vi "Img Plot Frame.vi"(8 "error in (no error)":errorcluster, 9 "frames":T2, 10 "Img Data indexed":cluster{"image data":T1, "bitmap":u32[][]}, 11 "LF2R IDE in":refnum<class "Main Panel.lvclass">) -> (0 "error out":errorcluster, 3 "LF2R IDE out":refnum<class "Main Panel.lvclass">)   [LabVIEW 2018, in "Main Panel.lvlib" / "Main Panel.lvclass"]
uses:
  Main Panel.lvclass
  Image Json Parser/Img Json Frames.ctl
  <vilib>/picture/picture.llb/imagedata.ctl
  Main Panel.lvclass/Main Panel.ctl
  <vilib>/picture/picture.llb/Draw True-Color Pixmap.vi
  Picture Process/Picture Process.lvclass
  Image Json Parser/Image Json Parser.lvclass
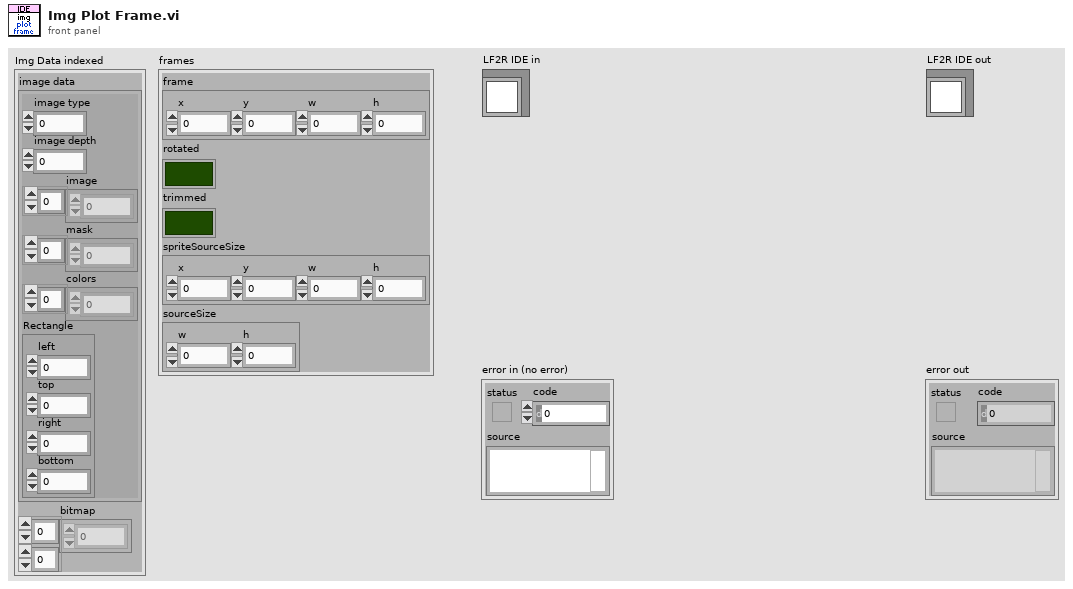
[diagram p1: front panel]
types:
  T1 = typedef "imagedata.ctl" = cluster{"image type":i32, "image depth":i32, "image":u8[], "mask":u8[], "colors":u32[], "Rectangle":cluster{"left":i16, "top":i16, "right":i16, "bottom":i16}}
  T2 = typedef "Image Json Parser.lvclass/Img Json Frames.ctl" = cluster{"frame":cluster{"x":i32, "y":i32, "w":i32, "h":i32}, "rotated":bool, "trimmed":bool, "spriteSourceSize":cluster{"x":i32, "y":i32, "w":i32, "h":i32}, "sourceSize":cluster{"w":i32, "h":i32}}
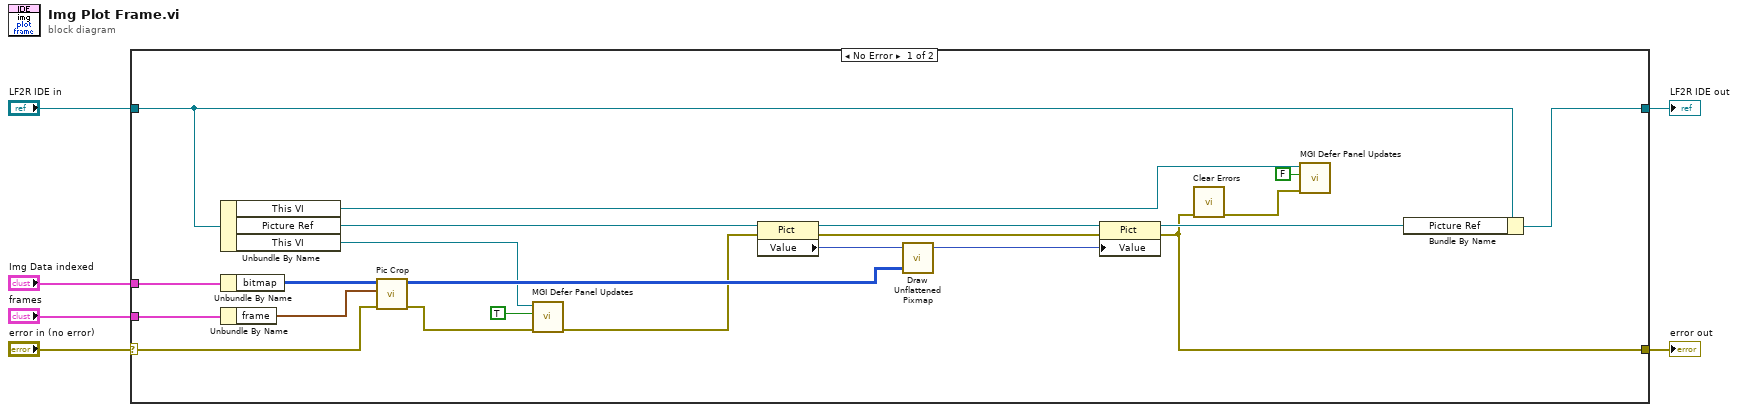
[diagram p0: block diagram]
diagram:
  n1 = case shown="No Error" "error in (no error)" {
    selector: "error in (no error)" -> [w11 w30]
    tunnel: [w7 w30] -> w5
    tunnel: [w25 w29] -> w3
    tunnel: "LF2R IDE in" -> [w26 w29]
    tunnel: "Img Data indexed" -> [w28 _]
    tunnel: "frames" -> [w27 _]
    frame No Error {
      n2 = Unbundle By Name(w26) -> ("This VI"=w10:refnum<vi>, "Picture Ref"=w24:refnum<vi>, "This VI"=w13:refnum<vi>)
      n3 = Unbundle By Name(w28) -> ("bitmap"=w23:u32[][])
      n4 = Unbundle By Name(w27) -> ("frame"=w20:cluster{"x":i32, "y":i32, "w":i32, "h":i32})
      n5 = call "Pic Crop.vi"("error in (no error)"=w11, "Position"=w20, "24-bit pixmap in"=w23) -> ("error out"=w15:errorcluster, "24-bit pixmap out"=w21:u32[][])  [unwired: 7 in]
      n6 = call <userlib>:"MGI Defer Panel Updates.vi"("Error In"=w15, "Defer Updates?"=TRUE, "VI Reference (Caller)"=w13) -> ("Error Out"=w14:errorcluster)  [unwired: 8 in]
      n7 = property class="Pict"(reference=w24, error in=w14) -> (reference out=w19:refnum<vi>, error out=w18:errorcluster, "Value"=w22:picture)
      n8 = call-poly <vilib>:"Draw Unflattened Pixmap.vi"("picture"=w22, "data (RGB format)"=w21) -> ("new picture"=w17:picture)  [unwired: 7 in]
      n9 = property class="Pict"(reference=w19, error in=w18, "Value"=w17) -> (reference out=w16:refnum<vi>, error out=w7:errorcluster)
      n10 = call <vilib>:"Clear Errors.vi"("error in (no error)"=w7) -> ("error out"=w8:errorcluster)  [unwired: 5 in, 1 out]
      n11 = call <userlib>:"MGI Defer Panel Updates.vi"("Error In"=w8, "Defer Updates?"=FALSE, "VI Reference (Caller)"=w10) -> ()  [unwired: 8 in, 1 out]
      n12 = Bundle By Name(cluster=w26, "Picture Ref"=w16) -> (w25:refnum<class "Main Panel.lvclass">)
    }
    frame Error {
    }
  }
  "error out" <- w5
  "LF2R IDE out" <- w3
